vi "pixel_to_energy.vi"(0 "Calibration Data":cluster{"quad_term":dbl, "linear_term":dbl}, 1 "PES Data In":cluster{"Pixel":dbl[], "Intensity":dbl[]}, 7 "Detachment Wavelength / nm":dbl, 11 "error in":errorcluster) -> (3 "PES Data Out":T1, 15 "error out":errorcluster)   [LabVIEW 2023]
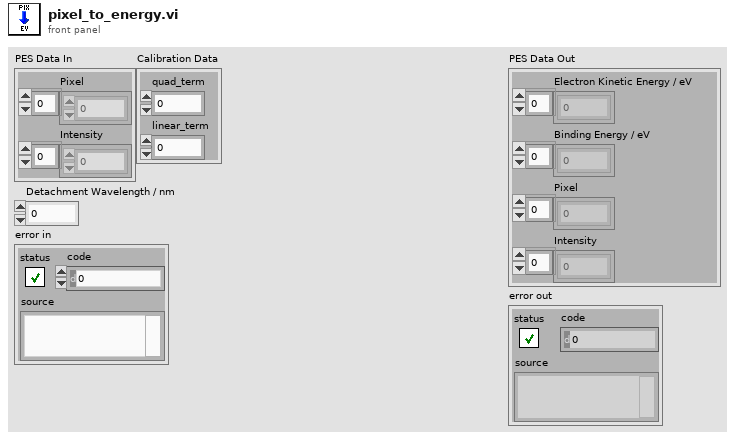
[diagram p1: front panel]
types:
  T1 = cluster{"Electron Kinetic Energy / eV":dbl[], "Binding Energy / eV":dbl[], "Pixel":dbl[], "Intensity":dbl[]}
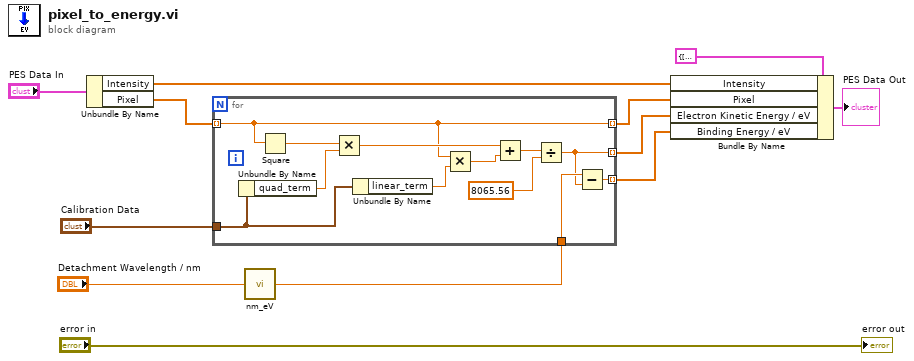
[diagram p0: block diagram]
diagram:
  n1 = Unbundle By Name("PES Data In") -> ("Intensity"=w3:dbl[], "Pixel"=w9:dbl[])
  n2 = call "nm_eV.vi"("nm"="Detachment Wavelength / nm") -> ("eV"=w5:dbl)  [unwired: 14 in]
  n3 = for {
    tunnel: "Calibration Data" -> [w22]
    tunnel: w9 -> [w16] mode=indexing
    tunnel: [w14] -> w7 mode=indexing
    tunnel: [w16] -> w8 mode=indexing
    tunnel: w5 -> [w15]
    tunnel: [w13] -> w4 mode=indexing
    n4 = Unbundle By Name(w22) -> ("quad_term"=w24:dbl)
    n5 = Square(x=w16) -> (x^2=w23:dbl)
    n6 = Multiply(x=w23, y=w24) -> (x*y=w20:dbl)
    n7 = Unbundle By Name(w22) -> ("linear_term"=w21:dbl)
    n8 = Multiply(x=w16, y=w21) -> (x*y=w19:dbl)
    n9 = Add(x=w20, y=w19) -> (x+y=w18:dbl)
    n10 = Divide(x=w18, y=8065.56) -> (x/y=w14:dbl)
    n11 = Subtract(x=w15, y=w14) -> (x-y=w13:dbl)
  }
  n12 = Bundle By Name(cluster=T1 {"Electron Kinetic Energy / eV"=[], "Binding Energy / eV"=[], "Pixel"=[], "Intensity"=[]}, "Intensity"=w3, "Pixel"=w8, "Electron Kinetic Energy / eV"=w7, "Binding Energy / eV"=w4) -> (→"PES Data Out":T1)
  "error out" <- "error in"
